vi "Calc Channel Query.vi"(8 "error in":errorcluster, 10 "Channel":i32(ring) caption="Calculation Channel" items=["Calc Channel 1", "Calc Channel 2", "Calc Channel 3", "Calc Channel 4"], 11 "Instrument Handle In":i32) -> (0 "error out":errorcluster, 2 "State":i32, 3 "Instrument Handle Out":i32)   [LabVIEW 8.6, in "ZTScopeM.lvlib"]
doc: "Query the state of the selected calculation channel."
uses:
  ZTScopeM.lvlib
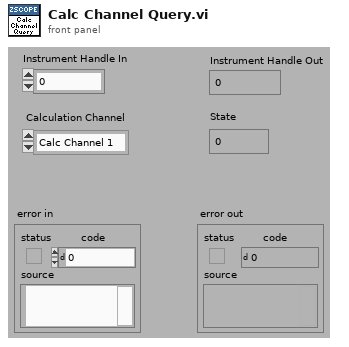
[diagram p1: front panel]
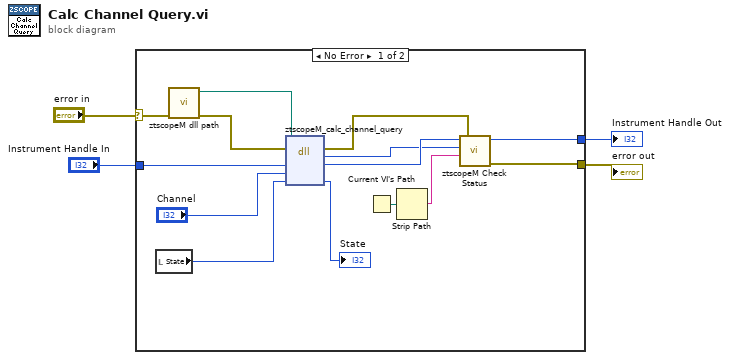
[diagram p0: block diagram]
diagram:
  n1 = case shown="No Error" "error in" {
    selector: "error in" -> [w8 w20]
    tunnel: [w9 w20] -> w1
    tunnel: "Instrument Handle In" -> [w18 w19]
    tunnel: [w10 w19] -> w3
    frame #0 {
      n2 = local read "State"() -> (w16:i32)
      n3 = call "ztscopeM dll path.vi"("error in (no error)"=w8) -> ("error out"=w6:errorcluster, "<instrument>.dll path"=w7:path)  [unwired: 9 in]
      n4 = dll-call lib="C:/Program Files (x86)/National Instruments/LabVIEW 2013/instr.lib/ztscopem/ztscopeM.dll" fn="ztscopeM_calc_channel_query"(path in=w7, error in=w6, "instrumentHandle"=w18, "calculationChannel"="Channel", "state"=w16) -> (error out=w5:errorcluster, w11:i32, "instrumentHandle"=w12:i32, "state"=→"State":i32)  [unwired: 2 in, 1 out]
      n5 = Current VI's Path() -> (path=w14:path)
      n6 = Strip Path(path=w14) -> (name=w13:string)  [unwired: 1 out]
      n7 = call "ztscopeM Check Status.vi"("error in"=w5, "name of VI"=w13, "status (return code)"=w11, "instrument handle in"=w12) -> ("error out"=w9:errorcluster, "instrument handle out"=w10:i32)  [unwired: 2 in]
    }
    frame #1 {
    }
  }
  "Instrument Handle Out" <- w3
  "error out" <- w1
